vi "Record Recent User.vi"(8 "error in (no error)":errorcluster, 10 "username":string, 11 "[C] User Management in":refnum<class "[C] User Management.lvclass">) -> (0 "error out":errorcluster, 3 "[C] User Management out":refnum<class "[C] User Management.lvclass">)   [LabVIEW 2020, in "[C] User Management.lvlib" / "[C] User Management.lvclass"]
uses:
  [C] User Management.lvclass
  [C] User Management.lvclass/[C] User Management.ctl
  213a1c76-b2bf-4534-87b1-10d592c3c6bd.vi
  <vilib>/Comparison/Equal/Equal Functor/Equal Functor.lvclass
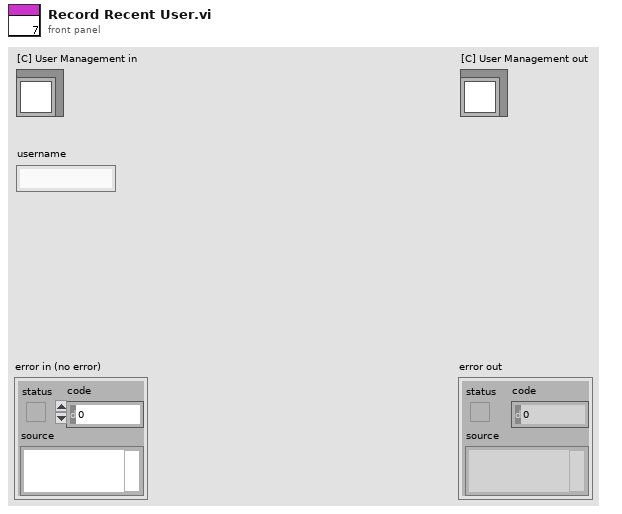
[diagram p1: front panel]
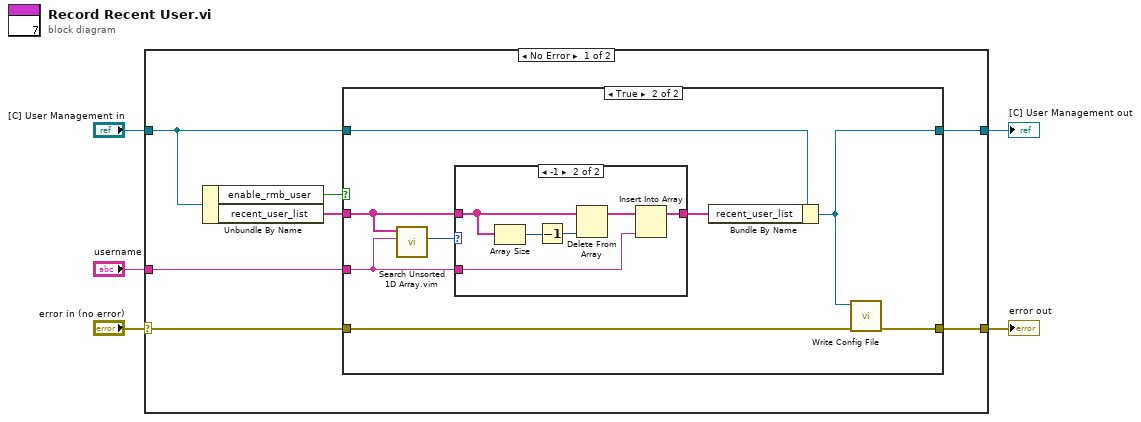
[diagram p0: block diagram]
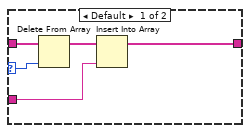
[diagram p3: hidden frame]
diagram:
  n1 = case shown="No Error" "error in (no error)" {
    selector: "error in (no error)" -> [w8 w35]
    tunnel: [w7 w35] -> w4
    tunnel: [w6 w34] -> w2
    tunnel: "[C] User Management in" -> [w9 w34]
    tunnel: "username" -> [w10 _]
    frame No Error {
      n2 = Unbundle By Name(w9) -> ("enable_rmb_user"=w12:bool, "recent_user_list"=w11:string[])
      n3 = case shown="True" w12 {
        tunnel: w11 -> [_ w21]
        tunnel: w10 -> [_ w20]
        tunnel: w9 -> [w14 w19]
        tunnel: w8 -> [w13 w17]
        tunnel: [w13 w16] -> w7
        tunnel: [w14 w15] -> w6
        frame False {
        }
        frame True {
          n4 = call "Search Unsorted 1D Array.vim"("element"=w20, "unsorted 1D array"=w21) -> ("index of element"=w22:i32)  [unwired: 9 in]
          n5 = case shown="-1" w22 {
            selector: w22 -> [w26 _]
            tunnel: w21 -> [w27 w33]
            tunnel: w20 -> [w24 w29]
            tunnel: [w23 w28] -> w18
            frame Default {
              n6 = Delete From Array(array=w27, index=w26) -> (array with subset deleted=w25:string[])  [unwired: 1 in, 1 out]
              n7 = Insert Into Array(array=w25, new element=w24) -> (w23:string[])  [unwired: 1 in]
            }
            frame -1 {
              n8 = Array Size(array=w33) -> (size(s)=w32:i32)
              n9 = Decrement(x=w32) -> (x-1=w31:i32)
              n10 = Delete From Array(array=w33, index=w31) -> (array with subset deleted=w30:string[])  [unwired: 1 in, 1 out]
              n11 = Insert Into Array(array=w30, new element=w29) -> (w28:string[])  [unwired: 1 in]
            }
          }
          n12 = Bundle By Name(cluster=w19, "recent_user_list"=w18) -> (w15:refnum<class "[C] User Management.lvclass">)
          n13 = call "Write Config File.vi"("error in (no error)"=w17, "[C] User Management in"=w15) -> ("error out"=w16:errorcluster)  [unwired: 8 in, 1 out]
        }
      }
    }
    frame Error {
    }
  }
  "error out" <- w4
  "[C] User Management out" <- w2
